vi "TestGlobal.vi"() -> ()   [LabVIEW 2013]
panel:
  out "Numerisch":u32
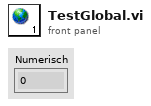
[diagram p1: front panel]
diagram:
